vi "Open Context.vi"(8 "error in (no error)":errorcluster, 11 "RemoteControl.ZMQ in":refnum<class "RemoteControl.ZMQ.lvclass">) -> (0 "error out":errorcluster, 3 "RemoteControl.ZMQ out":refnum<class "RemoteControl.ZMQ.lvclass">)   [LabVIEW 2020, in "RemoteControl.ZMQ.lvclass"]
uses:
  RemoteControl.ZMQ.lvclass
  RemoteControl.ZMQ.lvclass/RemoteControl.ZMQ.ctl
  <vilib>/addons/zeromq/zmq_context.lvclass
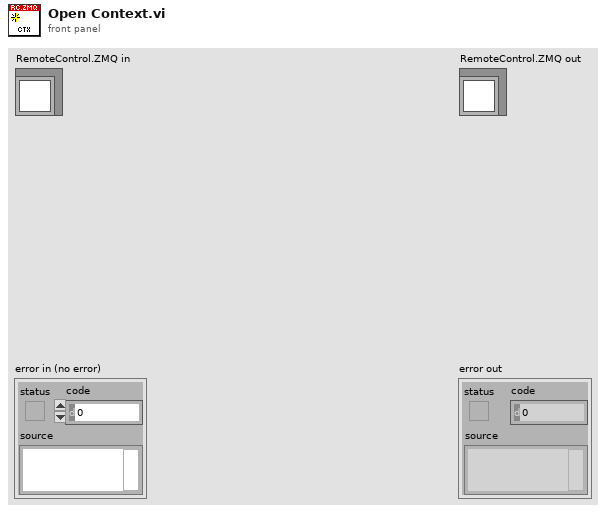
[diagram p1: front panel]
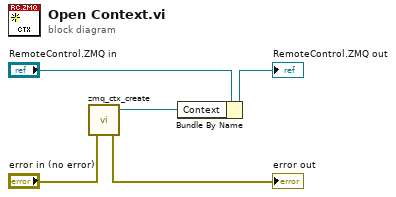
[diagram p0: block diagram]
diagram:
  n1 = call <vilib>:"zmq_ctx_create.vi"("error in"="error in (no error)") -> ("error out"=→"error out":errorcluster, "context out"=w3:refnum<class "zmq_context.lvclass">)  [unwired: 3 in]
  n2 = Bundle By Name(cluster="RemoteControl.ZMQ in", "Context"=w3) -> (→"RemoteControl.ZMQ out":refnum<class "RemoteControl.ZMQ.lvclass">)
